vi "PH_gentec_M-Link.get data to modify.vi"(0 "i ref in":refnum<vi>, 3 "ms timeout (10000)":i32=10000, 5 "error in (no error)":errorcluster) -> (14 "i ref out":refnum<vi>, 16 "i attribute":T1 {"Current Head Settings"."Waveform Averages" items=["None", "2", "4", "8", "16", "32", "64", "128"]; "Current Head Settings"."Trigger Source" items=["Internal", "External"]; "Current Head Settings"."Trigger Polarity" items=["Falling Edge", "Rising Edge"]; "Current Head Settings"."Measurement Mode" items=["other Mode", "Energymode"]; "Wanted Head Settings"."Waveform Averages" items=["None", "2", "4", "8", "16", "32", "64", "128"]; "Wanted Head Settings"."Trigger Source" items=["Internal", "External"]; "Wanted Head Settings"."Trigger Polarity" items=["Falling Edge", "Rising Edge"]; "Wanted Head Settings"."Measurement Mode" items=["other Mode", "Energymode"]}, 17 "timed out":bool, 19 "error out":errorcluster)   [LabVIEW 2014, in "PH_gentec_M-Link.lvlib"]
doc: "Reads the attribute data of the object after the access to the data has been locked by the \"acquire\" method. If the attribute data has been locked already, this methods waits until the attribute data is unlocked or there is a timeout.\n\nThe attribute data must be unlocked using the methods \"release\" or \"set modified data\".\n\nLicense Agreement for this software:\n\nCopyright (C)\nGesellschaft für Schwerionenforschung, GSI\nPlanckstr. 1\n64291 Darmstadt\nGermany\n\nContact: D.Beck@gsi.de \n\nThis program is free software; you can redistribute it and/or modify it under the terms of the GNU General Public License as published by the Free Software Foundation; either version 2 of the license, or (at your option) any later version.\n\nThis program is distributed in the hope that it will be useful, but WITHOUT ANY WARRANTY; without even the implied warranty of MERCHANTABILITY or FITNESS FOR A PARTICULAR PURPOSE. See the GNU General License for more details (http://www.gnu.org).\n\nGesellschaft für Schwerionenforschung, GSI\nPlanckstr. 1, 64291 Darmstadt, Germany\nFor all questions and ideas contact: M.Richter@gsi.de, H.Brand@gsi.de or D.Beck@gsi.de.\nLast update: 17-JUN-2004"
uses:
  PH_gentec_M-Link.lvlib
  PH_gentec_M-Link.i attribute.ctl
  PH_gentec_M-Link.Head Settings.ctl
  instr.lib/Gentec-M-Link/Driver/Type Defs/gentec-M-Link.Measurement Mode.ctl
  instr.lib/Gentec-M-Link/Driver/Type Defs/gentec-M-Link.Trigger Polarity.ctl
  instr.lib/Gentec-M-Link/Driver/Type Defs/gentec-M-Link.Trigger Source.ctl
  instr.lib/Gentec-M-Link/Driver/Type Defs/gentec-M-Link.Waveform Averages.ctl
  CS_Core/CSObj/CSObj.lvlib
  instr.lib/Gentec-M-Link/gentec-M-Link - Driver.lvlib
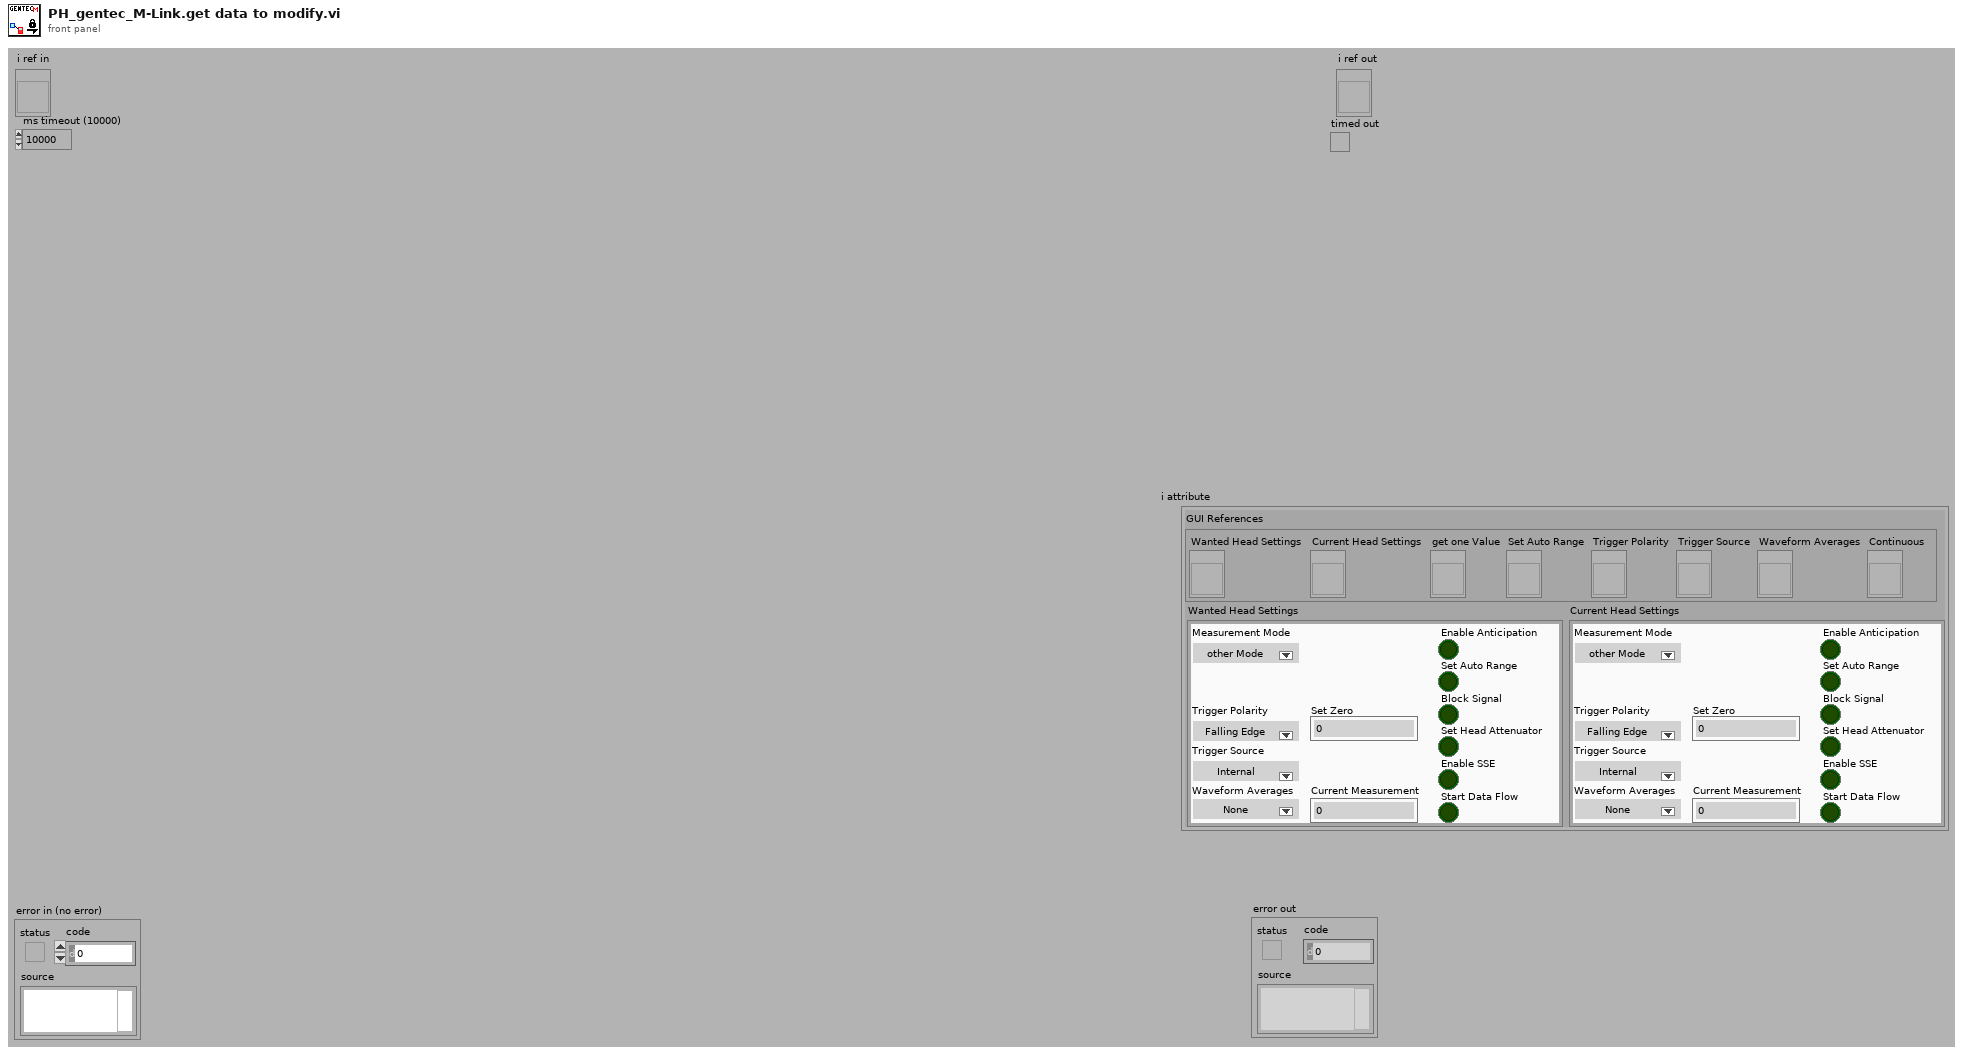
[diagram p1: front panel]
types:
  T1 = typedef "PH_gentec_M-Link.lvlib/PH_gentec_M-Link.i attribute.ctl" = cluster{"GUI References":cluster{"Wanted Head Settings":refnum<vi>, "Current Head Settings":refnum<vi>, "Set Auto Range":refnum<vi>, "Trigger Polarity":refnum<vi>, "Trigger Source":refnum<vi>, "Waveform Averages":refnum<vi>, "Continuous":refnum<vi>, "get one Value":refnum<vi>}, "Wanted Head Settings":T2, "Current Head Settings":T2}
  T2 = typedef "PH_gentec_M-Link.lvlib/PH_gentec_M-Link.Head Settings.ctl" = cluster{"Measurement Mode":T3, "Enable Anticipation":bool, "Set Auto Range":bool, "Block Signal":bool, "Set Head Attenuator":bool, "Enable SSE":bool, "Trigger Polarity":T4, "Trigger Source":T5, "Waveform Averages":T6, "Set Zero":i32, "Current Measurement":i32, "Start Data Flow":bool}
  T3 = typedef "gentec-M-Link - Driver.lvlib/gentec-M-Link.Measurement Mode.ctl" = u16
  T4 = typedef "gentec-M-Link - Driver.lvlib/gentec-M-Link.Trigger Polarity.ctl" = u16
  T5 = typedef "gentec-M-Link - Driver.lvlib/gentec-M-Link.Trigger Source.ctl" = u16
  T6 = typedef "gentec-M-Link - Driver.lvlib/gentec-M-Link.Waveform Averages.ctl" = u16
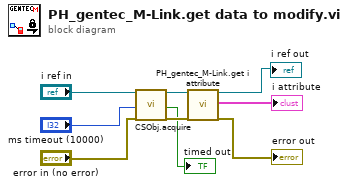
[diagram p0: block diagram]
diagram:
  n1 = call "CSObj.acquire.vi"("i ref in"="i ref in", "ms timeout (10000)"="ms timeout (10000)", "error in (no error)"="error in (no error)") -> ("i ref out"=w8:refnum<vi>, "timed out"=→"timed out":bool, "error out"=w5:errorcluster)  [unwired: 14 in]
  n2 = call "PH_gentec_M-Link.get i attribute.vi"("i ref in"=w8, "error in (no error)"=w5) -> ("i ref out"=→"i ref out":refnum<vi>, "i attribute"=→"i attribute":T1, "error out"=→"error out":errorcluster)  [unwired: 15 in]
